vi "Update Path Nodes.vi"(8 "error in (no error)":errorcluster, 9 "New Paths Array":T1[](array[typedef]), 10 "Current Version in":string, 11 ".NET Refnum in":refnum<k24>) -> (0 "error out":errorcluster, 2 "Current Version out":string, 3 ".NET Refnum out":refnum<k24>)   [LabVIEW 2019, in "Instrument Addon System Explorer.lvlib"]
uses:
  Instrument Addon System Explorer.lvlib
  NationalInstruments.VeriStand.SystemStorage
  <vilib>/NI VeriStand/Custom Device API/Path Type.ctl
  <vilib>/NI VeriStand/Custom Device API/Custom Device API.lvlib
  <vilib>/NI VeriStand/Custom Device API/Path Specification.ctl
  <vilib>/NI VeriStand/Custom Device API/Custom Device Supported Target.ctl
  <vilib>/NI VeriStand/Custom Device API/Custom Device Path Data.ctl
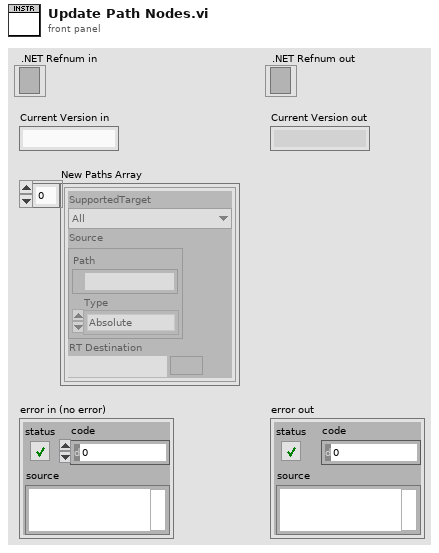
[diagram p1: front panel]
types:
  T1 = typedef "Custom Device API.lvlib/Custom Device Path Data.ctl" = cluster{"SupportedTarget":T2, "Source":T3, "RT Destination":path}
  T2 = typedef "Custom Device API.lvlib/Custom Device Supported Target.ctl" = enum16{"All", "PharLap", "VxWorks", "Windows", "Linux_32_ARM", "Linux_x64", "PharLap & Windows", "PharLap & VxWorks", "VxWorks & Windows"}
  T3 = typedef "Custom Device API.lvlib/Path Specification.ctl" = cluster{"Path":path, "Type":T4}
  T4 = typedef "Custom Device API.lvlib/Path Type.ctl" = enum16{"Absolute", "To Base", "To Common Data Dir", "To Application Data Dir"}
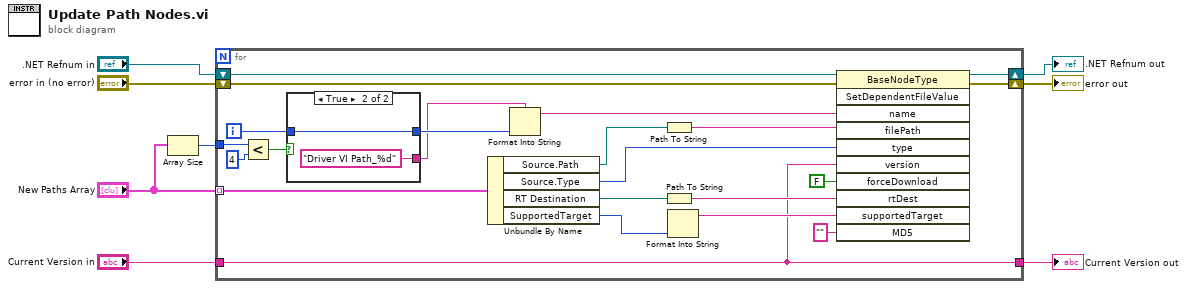
[diagram p0: block diagram]
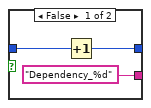
[diagram p2: hidden frame]
diagram:
  n1 = Array Size(array="New Paths Array") -> (size(s)=w1:i32)
  n2 = for {
    shift-right: [w27] -> w5
    shift-left: "error in (no error)" -> [w30]
    shift-right: [w28] -> w4
    shift-left: ".NET Refnum in" -> [w29]
    tunnel: "New Paths Array" -> [w26] mode=indexing
    tunnel: "Current Version in" -> [w15]
    tunnel: [w15] -> w7
    tunnel: w1 -> [w14]
    i -> [w11]
    n3 = Less?(x=w14, y=4) -> (x < y?=w12:bool)
    n4 = case shown="True" w12 {
      tunnel: w11 -> [w33 w35]
      tunnel: [w32 w35] -> w10
      tunnel: ["Dependency_%d" "Driver VI Path_%d"] -> w9
      frame False {
        n5 = Increment(x=w33) -> (x+1=w32:i32)
      }
      frame True {
      }
    }
    n6 = Unbundle By Name(w26) -> ("Source.Path"=w19:path, "Source.Type"=w24:T4, "RT Destination"=w18:path, "SupportedTarget"=w21:T2)
    n7 = Format Into String(format string=w9, w10) -> (resulting string=w25:string)  [unwired: 2 in, 1 out]
    n8 = Path To String(path=w19) -> (string=w16:string)
    n9 = Path To String(path=w18) -> (string=w17:string)
    n10 = Format Into String(w21) -> (resulting string=w20:string)  [unwired: 3 in, 1 out]
    n11 = invoke class="BaseNodeType" method="SetDependentFileValue"(reference=w29, error in=w30, "name"=w25, "filePath"=w16, "type"=w24, "version"=w15, "forceDownload"=FALSE, "rtDest"=w17, "supportedTarget"=w20, "MD5"="") -> (reference out=w28:refnum<k24>, error out=w27:errorcluster)  [unwired: 1 in, 9 out]
  }
  "Current Version out" <- w7
  "error out" <- w5
  ".NET Refnum out" <- w4
